vi "Loop Async.vi"(11 "AsyncClassTemplate in":refnum<class "AsyncClassTemplate.lvclass">) -> ()   [LabVIEW 2020, in "Vecto.lvlib" / "AsyncClassTemplate.lvclass"]
uses:
  AsyncClassTemplate.lvclass
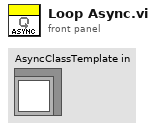
[diagram p1: front panel]
types:
  T1 = typedef "Vecto.lvlib/AsyncClassTemplate.lvclass/Loop Data.ctl" = cluster{"String":string}
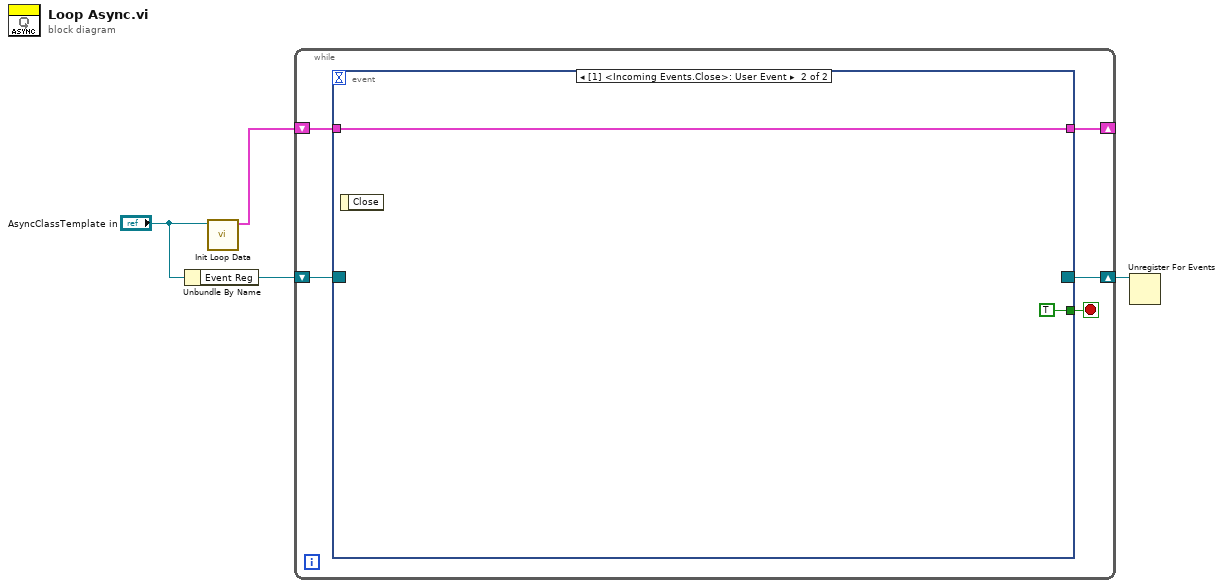
[diagram p0: block diagram]
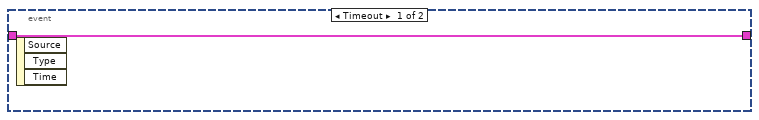
[diagram p2: hidden frame]
diagram:
  n1 = Unbundle By Name("AsyncClassTemplate in") -> ("Event Reg"=w4:refnum<event-registration>)
  n2 = call "Init Loop Data.vi"("AsyncClassTemplate in"="AsyncClassTemplate in") -> ("Loop Data"=w1:T1)  [unwired: 9 in, 1 out]
  n3 = while {
    shift-right: [w8] -> w3
    shift-left: w4 -> [w9]
    shift-right: [w5] -> _
    shift-left: w1 -> [w6]
    stop <- w7 stop-if-true
    n4 = event shown="[1] <Incoming Events.Close>: User Event" {
      selector: w9 -> [_ _]
      dyn-events: [_ _] -> w8
      timeout: _ -> [_ _]
      tunnel: [_ TRUE] -> w7
      tunnel: w6 -> [w10 w11]
      tunnel: [w10 w11] -> w5
      event Timeout {
        n5 = event-data() -> ()  [unwired: 1 in, 3 out]
      }
      event User Event {
        n6 = event-data() -> ()  [unwired: 1 in, 1 out]
      }
    }
  }
  n7 = Unregister For Events(event registration refnum=w3) -> ()  [unwired: 1 in, 1 out]
